vi "Check.vi"(9 "log line":string, 10 "current file":refnum<file>, 11 "RolloverTrigger in":refnum<class "RolloverTrigger.lvclass">) -> (2 "rollover?":bool, 3 "RolloverTrigger out":refnum<class "RolloverTrigger.lvclass">)   [LabVIEW 2018, in "GLog.lvlib" / "RolloverTrigger.lvclass"]
doc: "Checks if the configured rollover condition has been met."
uses:
  RolloverTrigger.lvclass
panel:
  # "Connector Pane"
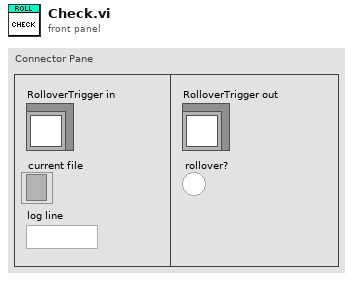
[diagram p1: front panel]
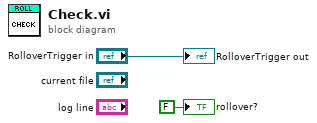
[diagram p0: block diagram]
diagram:
  "rollover?" <- FALSE ("rollover?")
  "RolloverTrigger out" <- "RolloverTrigger in"
